vi "Lookup Channel Indices by Name.vi"(8 "error in (no error)":errorcluster, 10 "Channel Names":string[](array[string]), 11 "Group in":refnum<class "Group Config.lvclass">) -> (0 "error out":errorcluster, 2 "Indices":i32[](array[numeric]), 3 "Group out":refnum<class "Group Config.lvclass">)   [LabVIEW 2020, in "VolatusConfig.lvlib" / "Group Config.lvclass"]
uses:
  Group Config.lvclass
  C:/dev/lv20CE/relink/lv-volatus/VolatusConfig/VolatusConfigElement/VolatusConfigElement.lvclass
  VolatusConfigElement/VolatusConfigElement.lvclass/VolatusConfigElement.ctl
  VolatusConfigElement/Element.vi
  Channel/Channel Config.lvclass
  Group Config.lvclass/Group Config.ctl
  VolatusConfigElement/VolatusConfigElement.lvclass
  C:/dev/lv20CE/relink/lv-volatus/VolatusConfig/Channel/Channel Config.lvclass
  C:/dev/lv20CE/relink/lv-volatus/VolatusConfig/Group/Group Config.lvclass
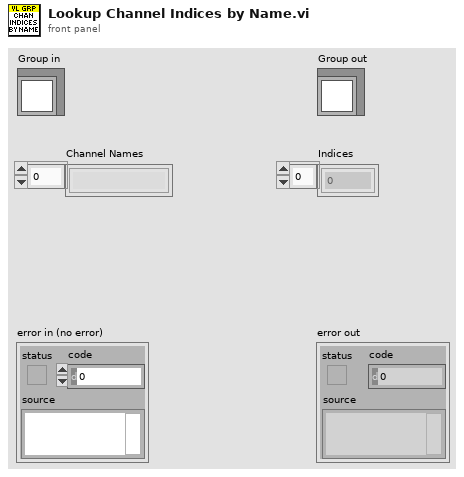
[diagram p1: front panel]
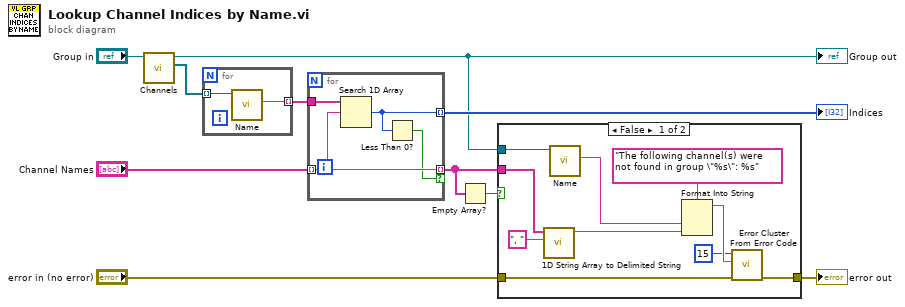
[diagram p0: block diagram]
diagram:
  n1 = call "Channels.vi"("Group in"="Group in") -> ("Channels"=w8:refnum<class "Channel Config.lvclass">[], "Group out"=w1:refnum<class "Group Config.lvclass">)  [unwired: 8 in, 1 out]
  "Group out" <- w1
  n2 = for {
    tunnel: w8 -> [w12] mode=indexing
    tunnel: [w11] -> w7 mode=indexing
    n3 = call "Name.vi"("VolatusConfigElement in"=w12) -> ("Name"=w11:string)  [unwired: 8 in, 2 out]
  }
  n4 = for {
    tunnel: w7 -> [w16]
    tunnel: "Channel Names" -> [w15] mode=indexing
    tunnel: [w15] -> w2 mode=indexing if=w13
    tunnel: [w14] -> w5 mode=indexing
    n5 = Search 1D Array(1D array=w16, element=w15) -> (index of element=w14:i32)  [unwired: 1 in]
    n6 = Less Than 0?(x=w14) -> (x < 0?=w13:bool)
  }
  "Indices" <- w5
  n7 = Empty Array?(array=w2) -> (empty?=w3:bool)
  n8 = case shown="False" w3 {
    tunnel: "error in (no error)" -> [w26 w27]
    tunnel: [w25 w27] -> w4
    tunnel: w2 -> [w24 _]
    tunnel: w1 -> [w22 _]
    frame False {
      n9 = call <vilib>:"1D String Array to Delimited String.vi"("delimiter"=", ", "string array"=w24) -> ("delimited string"=w18:string)  [unwired: 9 in]
      n10 = call "Name.vi"("VolatusConfigElement in"=w22) -> ("Name"=w17:string)  [unwired: 8 in, 2 out]
      n11 = Format Into String(format string="The following channel(s) were not found in group \"%s\": %s", w17, w18) -> (resulting string=w20:string)  [unwired: 2 in, 1 out]
      n12 = call <vilib>:"Error Cluster From Error Code.vi"("error in (no error)"=w26, "error message (\"\")"=w20, "error code (0)"=15) -> ("error out"=w25:errorcluster)  [unwired: 6 in]
    }
    frame True {
    }
  }
  "error out" <- w4
